vi "poly_data_queue_double.vi"(6 "initial queue element (NaN)":dbl=nan, 7 "initialize":bool, 8 "Error in":errorcluster caption="Error in (no error)", 10 "sample length":i32=100, 11 "input data point":dbl format="%0.2f") -> (0 "Error out":errorcluster, 2 "Queue":dbl[](array[numeric]), 3 "eliminated element":dbl format="%0.2f", 4 "current length":i32)   [LabVIEW 2015, in "_average_tools_polys.lvlib"]
uses:
  _average_tools_polys.lvlib
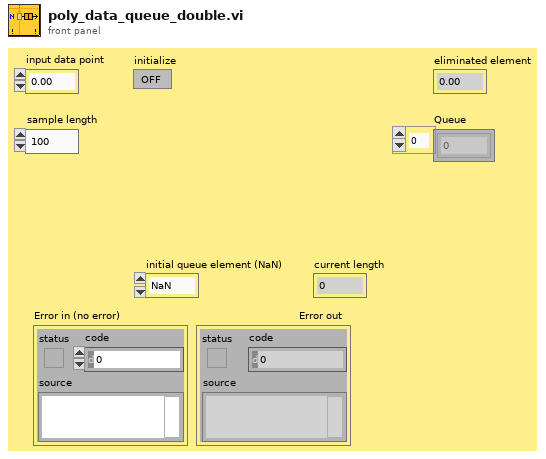
[diagram p1: front panel]
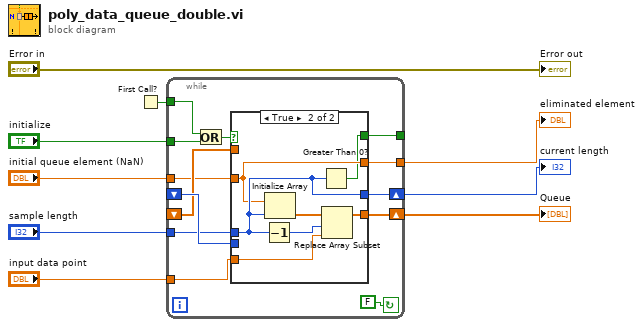
[diagram p0: block diagram]
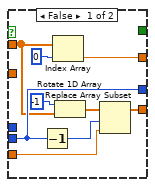
[diagram p2: hidden frame]
diagram:
  n1 = First Call?() -> (First Call?: T/F=w7:bool)
  n2 = while {
    tunnel: w7 -> [w17]
    shift-left: _ -> [w20]
    shift-right: [w21] -> w8
    shift-left: _ -> [w19]
    shift-right: [w22] -> w9
    tunnel: "initialize" -> [w15]
    tunnel: "input data point" -> [w14]
    tunnel: "initial queue element (NaN)" -> [w13]
    tunnel: "sample length" -> [w12]
    tunnel: [w11] -> w2
    tunnel: [w10] -> _
    stop <- FALSE continue-if-true
    n3 = Or(x=w17, y=w15) -> (x .or. y?=w16:bool)
    n4 = case shown="True" w16 {
      tunnel: [w28 w34] -> w22
      tunnel: [w29 w37] -> w21
      tunnel: w20 -> [w29 _]
      tunnel: w19 -> [w25 _]
      tunnel: w14 -> [w30 w35]
      tunnel: w13 -> [_ w33]
      tunnel: w12 -> [_ w37]
      tunnel: [w23 w33] -> w11
      tunnel: [_ w32] -> w10
      frame False {
        n5 = Decrement(x=w29) -> (x-1=w27:i32)
        n6 = Index Array(array=w25, index=0 ("Index")) -> (element=w23:dbl)
        n7 = Rotate 1D Array(1:w25, 2:i16 -1 ("n")) -> (0:w26:dbl[])
        n8 = Replace Array Subset(array=w26, new element=w30, index=w27) -> (w28:dbl[])
      }
      frame True {
        n9 = Decrement(x=w37) -> (x-1=w38:i32)
        n10 = Initialize Array(w33, w37) -> (w36:dbl[])
        n11 = Greater Than 0?(x=w37) -> (x > 0?=w32:bool)
        n12 = Replace Array Subset(array=w36, new element=w35, index=w38) -> (w34:dbl[])
      }
    }
  }
  "Queue" <- w9
  "current length" <- w8
  "eliminated element" <- w2
  "Error out" <- "Error in"
